vi "Initialize.vi"(8 "error in (no error)":errorcluster, 10 "Cal file":path, 11 "Level in":refnum<class "Level.lvclass">) -> (0 "error out":errorcluster, 3 "Level out":refnum<class "Level.lvclass">)   [LabVIEW 2020, in "Level.lvclass"]
uses:
  Level.lvclass
  Level.lvclass/Level.ctl
  <vilib>/regexp/Match Regular Expression.xnode
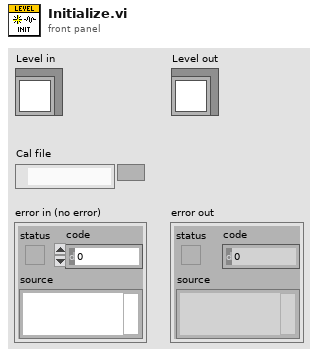
[diagram p1: front panel]
types:
  T1 = typedef "Level.lvclass/LevelUnits.ctl" = enum16{"dB atten", "dB SPL", "dB Vrms", "Volts", "dB mW", "mW", "dB HL", "dB SL"}
  T2 = typedef "LaserCal-Data (I-O).ctl" = cluster{"I-O":cluster{dbl[], dbl[]}, "Time-Domain":cluster{dbl[], dbl[]}[], "Time Index":i32, "Data header":string, "Tsettle (s)":dbl}
  T3 = typedef "LaserCal-Data (PT).ctl" = cluster{"I-O":cluster{"Volts":dbl[], "Width":dbl[], "Rate":dbl[], "Power":dbl[][][][]}, "Data header":string, "Tsettle (s)":dbl}
  T4 = cluster{"Volts":dbl[], "Width":dbl[], "Rate":dbl[], "Power":dbl[][][][]}
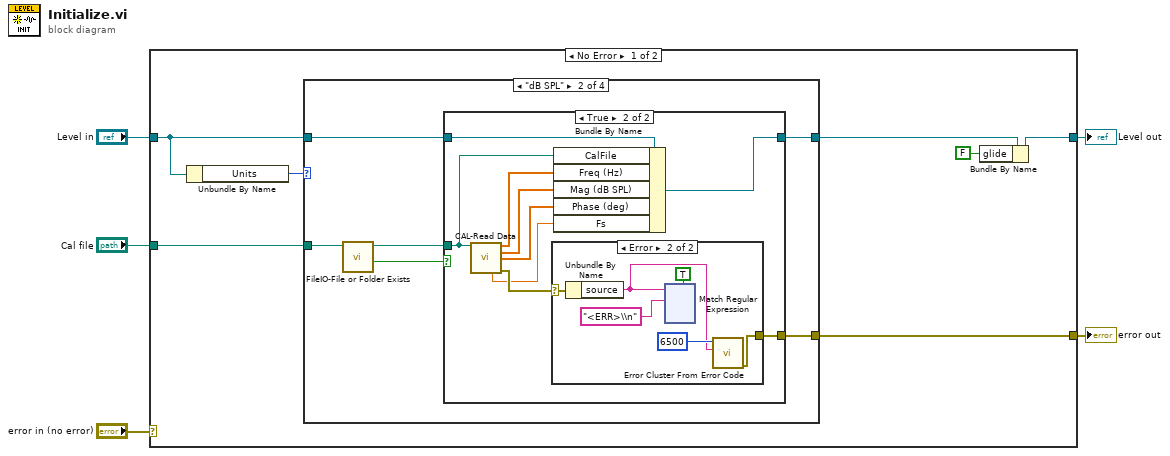
[diagram p0: block diagram]
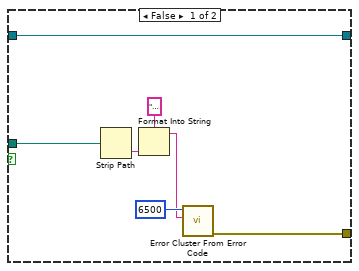
[diagram p3: hidden frame]
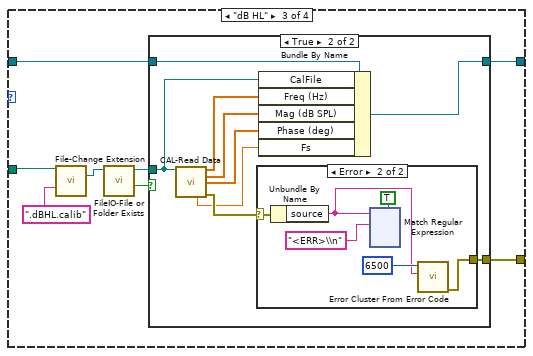
[diagram p5: hidden frame]
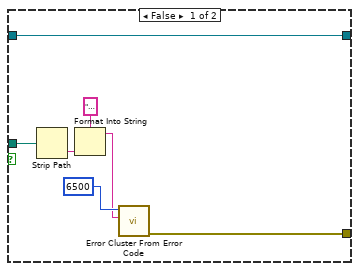
[diagram p6: hidden frame]
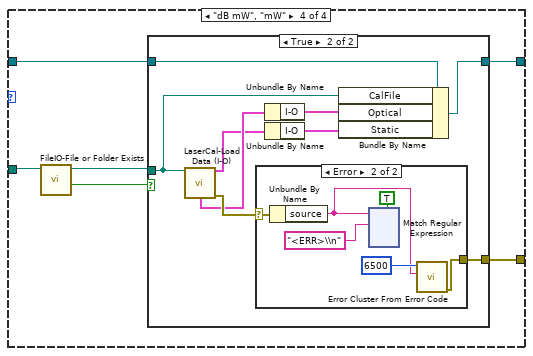
[diagram p8: hidden frame]
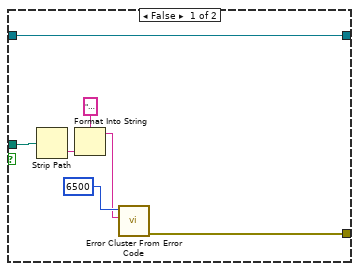
[diagram p9: hidden frame]
diagram:
  n1 = case shown="No Error" "error in (no error)" {
    selector: "error in (no error)" -> [_ w443]
    tunnel: [w9 w443] -> w4
    tunnel: [w7 w442] -> w2
    tunnel: "Level in" -> [w11 w442]
    tunnel: "Cal file" -> [w8 _]
    frame No Error {
      n2 = Unbundle By Name(w11) -> ("Units"=w12:T1)
      n3 = case shown="\"dB SPL\"" w12 {
        tunnel: w11 -> [w13 w18 w162 w305]
        tunnel: [w13 w17 w161 w304] -> w10
        tunnel: w8 -> [_ w16 w158 w302]
        tunnel: [_ w19 w163 w303] -> w9
        frame "dB atten", Default {
        }
        frame "dB SPL" {
          n4 = call "FileIO-File or Folder Exists.vi"("path"=w16) -> ("Exists?"=w14:bool, "dup path"=w15:path)  [unwired: 7 in, 2 out]
          n5 = case shown="True" w14 {
            tunnel: w15 -> [w26 w33]
            tunnel: [w25 w28] -> w19
            tunnel: w18 -> [w24 w35]
            tunnel: [w24 w34] -> w17
            frame False {
              n6 = Strip Path(path=w26) -> (name=w21:string)  [unwired: 1 out]
              n7 = Format Into String(format string="Calibration file '%s' was not found.", w21) -> (resulting string=w20:string)  [unwired: 2 in, 1 out]
              n8 = call <vilib>:"Error Cluster From Error Code.vi"("error message (\"\")"=w20, "error code (0)"=6500 ("specific error code to clear (0: all)")) -> ("error out"=w25:errorcluster)  [unwired: 7 in]
            }
            frame True {
              n9 = call "CAL-Read Data.vi"("user path"=w33) -> ("Frequency (Hz)"=w32:dbl[], "Mag"=w31:dbl[], "Phase"=w30:dbl[], "Fs (Hz)"=w27:dbl, "error out"=w29:errorcluster)  [unwired: 10 in]
              n10 = case shown="Error" w29 {
                selector: w29 -> [_ w41]
                tunnel: [_ w39] -> w28
                frame No Error {
                }
                frame Error {
                  n11 = Unbundle By Name(w41) -> ("source"=w36:string)
                  n12 = xnode "Match Regular Expression"("input string"=w36, "regular expression"="<ERR>\\n", "multiline? (F)"=TRUE) -> ()  [unwired: 3 in, 5 out]
                  n13 = call <vilib>:"Error Cluster From Error Code.vi"("error message (\"\")"=w36, "error code (0)"=6500 ("specific error code to clear (0: all)")) -> ("error out"=w39:errorcluster)  [unwired: 7 in]
                }
              }
              n14 = Bundle By Name(cluster=w35, "CalFile"=w33, "Freq (Hz)"=w32, "Mag (dB SPL)"=w31, "Phase (deg)"=w30, "Fs"=w27) -> (w34:refnum<class "Level.lvclass">)
            }
          }
        }
        frame "dB HL" {
          n15 = call "File-Change Extension.vi"("Path"=w158, "new extension"=".dBHL.calib") -> ("new path"=w157:path)  [unwired: 12 in, 1 out]
          n16 = call "FileIO-File or Folder Exists.vi"("path"=w157) -> ("Exists?"=w159:bool, "dup path"=w160:path)  [unwired: 7 in, 2 out]
          n17 = case shown="True" w159 {
            tunnel: w160 -> [w169 w177]
            tunnel: [w165 w172] -> w163
            tunnel: w162 -> [w164 w179]
            tunnel: [w164 w178] -> w161
            frame False {
              n18 = Strip Path(path=w169) -> (name=w167:string)  [unwired: 1 out]
              n19 = Format Into String(format string="Calibration file '%s' was not found.", w167) -> (resulting string=w166:string)  [unwired: 2 in, 1 out]
              n20 = call <vilib>:"Error Cluster From Error Code.vi"("error message (\"\")"=w166, "error code (0)"=6500 ("specific error code to clear (0: all)")) -> ("error out"=w165:errorcluster)  [unwired: 7 in]
            }
            frame True {
              n21 = call "CAL-Read Data.vi"("user path"=w177) -> ("Frequency (Hz)"=w176:dbl[], "Mag"=w175:dbl[], "Phase"=w174:dbl[], "Fs (Hz)"=w171:dbl, "error out"=w173:errorcluster)  [unwired: 10 in]
              n22 = case shown="Error" w173 {
                selector: w173 -> [_ w185]
                tunnel: [_ w184] -> w172
                frame No Error {
                }
                frame Error {
                  n23 = Unbundle By Name(w185) -> ("source"=w180:string)
                  n24 = xnode "Match Regular Expression"("input string"=w180, "regular expression"="<ERR>\\n", "multiline? (F)"=TRUE) -> ()  [unwired: 3 in, 5 out]
                  n25 = call <vilib>:"Error Cluster From Error Code.vi"("error message (\"\")"=w180, "error code (0)"=6500 ("specific error code to clear (0: all)")) -> ("error out"=w184:errorcluster)  [unwired: 7 in]
                }
              }
              n26 = Bundle By Name(cluster=w179, "CalFile"=w177, "Freq (Hz)"=w176, "Mag (dB SPL)"=w175, "Phase (deg)"=w174, "Fs"=w171) -> (w178:refnum<class "Level.lvclass">)
            }
          }
        }
        frame "dB mW", "mW" {
          n27 = call "FileIO-File or Folder Exists.vi"("path"=w302) -> ("Exists?"=w300:bool, "dup path"=w301:path)  [unwired: 7 in, 2 out]
          n28 = case shown="True" w300 {
            tunnel: w301 -> [w311 w318]
            tunnel: [w307 w319] -> w303
            tunnel: w305 -> [w306 w321]
            tunnel: [w306 w320] -> w304
            frame False {
              n29 = Strip Path(path=w311) -> (name=w309:string)  [unwired: 1 out]
              n30 = Format Into String(format string="Calibration file '%s' was not found.", w309) -> (resulting string=w308:string)  [unwired: 2 in, 1 out]
              n31 = call <vilib>:"Error Cluster From Error Code.vi"("error message (\"\")"=w308, "error code (0)"=6500 ("specific error code to clear (0: all)")) -> ("error out"=w307:errorcluster)  [unwired: 7 in]
            }
            frame True {
              n32 = call "LaserCal-Load Data (I-O).vi"("Path"=w318) -> ("I-O Data (static)"=w314:T2, "I-O Data"=w316:T3, "error out"=w317:errorcluster)  [unwired: 7 in, 5 out]
              n33 = case shown="Error" w317 {
                selector: w317 -> [_ w327]
                tunnel: [_ w325] -> w319
                frame No Error {
                }
                frame Error {
                  n34 = Unbundle By Name(w327) -> ("source"=w322:string)
                  n35 = xnode "Match Regular Expression"("input string"=w322, "regular expression"="<ERR>\\n", "multiline? (F)"=TRUE) -> ()  [unwired: 3 in, 5 out]
                  n36 = call <vilib>:"Error Cluster From Error Code.vi"("error message (\"\")"=w322, "error code (0)"=6500 ("specific error code to clear (0: all)")) -> ("error out"=w325:errorcluster)  [unwired: 7 in]
                }
              }
              n37 = Unbundle By Name(w316) -> ("I-O"=w315:T4)
              n38 = Unbundle By Name(w314) -> ("I-O"=w313:cluster{dbl[], dbl[]})
              n39 = Bundle By Name(cluster=w321, "CalFile"=w318, "Optical"=w315, "Static"=w313) -> (w320:refnum<class "Level.lvclass">)
            }
          }
        }
      }
      n40 = Bundle By Name(cluster=w10, "glide"=FALSE) -> (w7:refnum<class "Level.lvclass">)
    }
    frame Error {
    }
  }
  "error out" <- w4
  "Level out" <- w2
